vi "Read OOB RX.vi"(8 "error in (no error)":errorcluster, 11 "CIFCorePlugin in":refnum<class "CIFCorePlugin.lvclass">) -> (0 "error out":errorcluster, 3 "CIFCorePlugin out":refnum<class "CIFCorePlugin.lvclass">)   [LabVIEW 2021, in "CIFCorePlugin.lvclass"]
uses:
  CIFCorePlugin.lvclass
  OOB/OOB_Rx/CIFCoreOOB_Rx.lvclass
  Typedef/Energized States.ctl
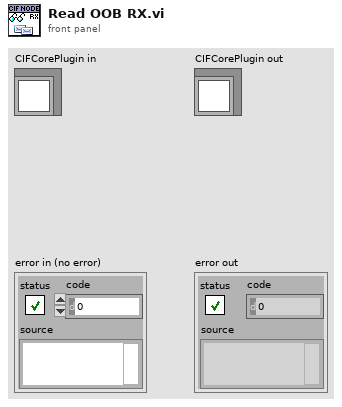
[diagram p1: front panel]
types:
  T1 = typedef "CIFCorePlugin.lvclass/Energized States.ctl" = enum16{"Listen", "Prepare", "Execute", "Housekeep", "Cleanup", "Destroy"}
  T2 = typedef "CIFCoreOOB_Rx.lvclass/OOB Core Commands.ctl" = enum8{"Start", "Pause", "Stop", "RefreshStats", "UpdateConfig", "Connect Channel", "Force Channel"}
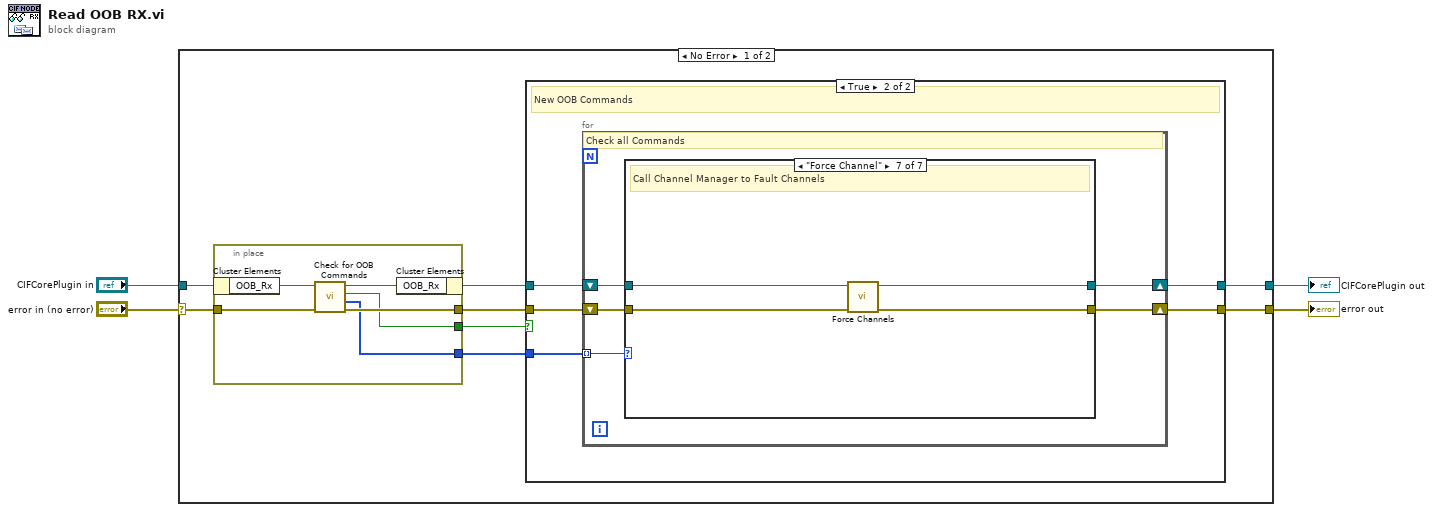
[diagram p0: block diagram]
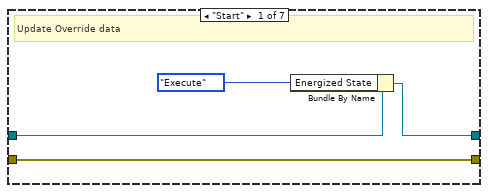
[diagram p3: hidden frame]
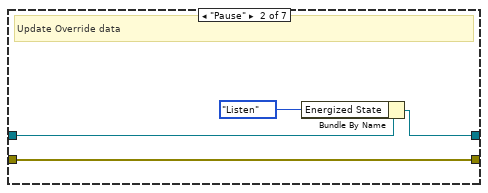
[diagram p4: hidden frame]
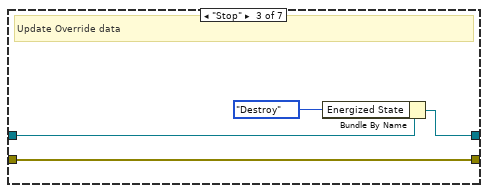
[diagram p5: hidden frame]
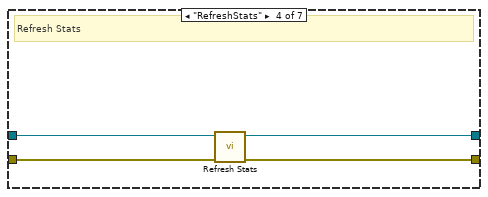
[diagram p6: hidden frame]
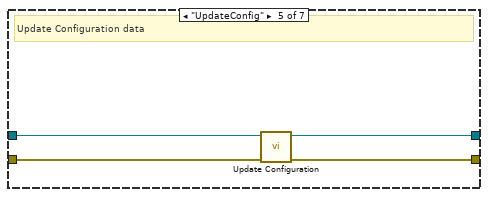
[diagram p7: hidden frame]
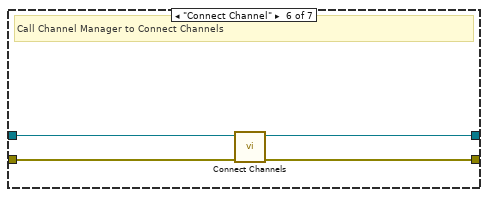
[diagram p8: hidden frame]
diagram:
  n1 = case shown="No Error" "error in (no error)" {
    selector: "error in (no error)" -> [w11 w60]
    tunnel: [w5 w60] -> w3
    tunnel: [w7 w59] -> w1
    tunnel: "CIFCorePlugin in" -> [w12 w59]
    frame No Error {
      n2 = in-place {
        in-place-border: w11 -> [w57]
        in-place-border: [w55] -> w6
        in-place-border: [w54] -> w9
        in-place-border: [w53] -> w10
        n3 = in-place-cluster #1(w12) -> ("OOB_Rx"=w58:refnum<class "CIFCoreOOB_Rx.lvclass">)
        n4 = call "Check for OOB Commands.vi"("error in (no error)"=w57, "CoreOOB_Rx in"=w58) -> ("error out"=w55:errorcluster, "Commands"=w54:T2[], "New Commands"=w53:bool, "CoreOOB_Rx out"=w56:refnum<class "CIFCoreOOB_Rx.lvclass">)  [unwired: 6 in]
        n5 = in-place-cluster #1("OOB_Rx"=w56) -> (w8:refnum<class "CIFCorePlugin.lvclass">)
      }
      n6 = case shown="True" w10 {
        tunnel: w9 -> [_ w19]
        tunnel: w8 -> [w14 w18]
        tunnel: [w14 w16] -> w7
        tunnel: w6 -> [w13 w17]
        tunnel: [w13 w15] -> w5
        frame False {
          # "No new OOB Commands"
        }
        frame True {
          # "New OOB Commands"
          n7 = for {
            tunnel: w19 -> [w24] mode=indexing
            shift-right: [w21] -> w16
            shift-left: w18 -> [w22]
            shift-right: [w20] -> w15
            shift-left: w17 -> [w23]
            # "Check all Commands"
            n8 = case shown="\"Force Channel\"" w24 {
              tunnel: w23 -> [w25 w32 w36 w39 w43 w47 w51]
              tunnel: w22 -> [w26 w31 w35 w40 w44 w48 w52]
              tunnel: [w28 w30 w34 w38 w42 w45 w50] -> w21
              tunnel: [w25 w32 w36 w37 w41 w46 w49] -> w20
              frame "Start" {
                # "Update Override data"
                n9 = Bundle By Name(cluster=w26, "Energized State"=Energized_States."Execute" ("Energized States in")) -> (w28:refnum<class "CIFCorePlugin.lvclass">)
              }
              frame "Pause" {
                # "Update Override data"
                n10 = Bundle By Name(cluster=w31, "Energized State"=Energized_States."Listen" ("Energized States in")) -> (w30:refnum<class "CIFCorePlugin.lvclass">)
              }
              frame "Stop" {
                # "Update Override data"
                n11 = Bundle By Name(cluster=w35, "Energized State"=Energized_States."Destroy" ("Energized States in")) -> (w34:refnum<class "CIFCorePlugin.lvclass">)
              }
              frame "RefreshStats" {
                # "Refresh Stats"
                n12 = call "Refresh Stats.vi"("error in (no error)"=w39, "CIFCorePlugin in"=w40) -> ("error out"=w37:errorcluster, "CIFCorePlugin out"=w38:refnum<class "CIFCorePlugin.lvclass">)  [unwired: 8 in]
              }
              frame "UpdateConfig" {
                # "Update Configuration data"
                n13 = call-dynamic "Update Configuration.vi"("error in (no error)"=w43, "CIFTemplateNode in"=w44) -> ("error out"=w41:errorcluster, "CIFTemplateNode out"=w42:refnum<class "CIFCorePlugin.lvclass">)  [unwired: 8 in]
              }
              frame "Connect Channel" {
                # "Call Channel Manager to Connect Channels"
                n14 = call "Connect Channels.vi"("error in (no error)"=w47, "CIFCorePlugin in"=w48) -> ("error out"=w46:errorcluster, "CIFCorePlugin out"=w45:refnum<class "CIFCorePlugin.lvclass">)  [unwired: 8 in]
              }
              frame "Force Channel" {
                # "Call Channel Manager to Fault Channels"
                n15 = call "Force Channels.vi"("error in (no error)"=w51, "CIFTemplateNode in"=w52) -> ("error out"=w49:errorcluster, "CIFTemplateNode out"=w50:refnum<class "CIFCorePlugin.lvclass">)  [unwired: 8 in]
              }
            }
          }
        }
      }
    }
    frame Error {
    }
  }
  "error out" <- w3
  "CIFCorePlugin out" <- w1
